vi "UseCaseDiagramGraph_Create.vi"(0 "reference":refnum<class "UseCaseDiagramGraph.lvclass">, 5 "error in (no error)":errorcluster) -> (14 "reference out":refnum<class "UseCaseDiagramGraph.lvclass">, 19 "error out":errorcluster)   [LabVIEW 2016, in "UseCaseDiagramGraph.lvclass"]
doc: "Creates and initializes a new UseCaseDiagramGraph object.\n\nThis object should be destroyed using a UseCaseDiagramGraph destructor VI or a virtual base class destructor VI.\n\n[GOOP 2.1]"
uses:
  <resource>/Framework/Providers/Open_GDS/UML/UseCaseDiagramGraph_class/UseCaseDiagramGraph.lvclass
  C:/Program Files (x86)/National Instruments/LabVIEW 2016/resource/Framework/Providers/Open_GDS/UML/Graph_class/Graph.lvclass
  <resource>/Framework/Providers/Open_GDS/UML/Graph_class/Graph.lvclass
panel:
  # "The input reference should only\nbe wired when this method is called\nby a sub class constructor."
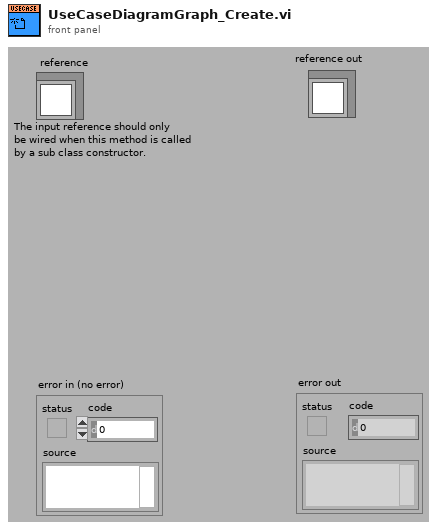
[diagram p1: front panel]
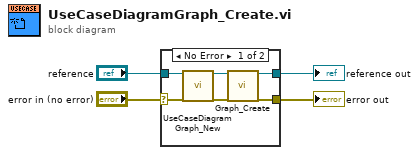
[diagram p0: block diagram]
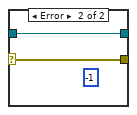
[diagram p2: hidden frame]
diagram:
  n1 = case shown="No Error" "error in (no error)" {
    selector: "error in (no error)" -> [w10 w12]
    tunnel: [w7 w11] -> w4
    tunnel: [w5 w12] -> w3
    tunnel: "reference" -> [w9 w11]
    frame No Error {
      n2 = call <resource>:"UseCaseDiagramGraph_New.vi"("reference in"=w9, "error in (no error)"=w10) -> ("reference out"=w8:refnum<class "UseCaseDiagramGraph.lvclass">, "error out"=w6:errorcluster)  [unwired: 2 in, 14 out]
      n3 = call <resource>:"Graph_Create.vi"("reference"=w8, "error in (no error)"=w6) -> ("reference out"=w7:refnum<class "UseCaseDiagramGraph.lvclass">, "error out"=w5:errorcluster)  [unwired: 1 in, 15 out]
    }
    frame Error {
      (unwired) -1 ("Nr of open handles")
    }
  }
  "error out" <- w3
  "reference out" <- w4
